vi "UTIL Initialize Median Filter.vi"(8 "Error In":errorcluster, 11 "Window Width":i32=60) -> (0 "Error Out":errorcluster, 3 "Average Queue":refnum<queue>)   [LabVIEW 2010]
doc: "Initialize a Moving Window Average routine by creating a fixed-length, Windows-sized Queue of Dbls, and initializing them to 0.\n\nInput:\n Window Size I32, default 10\n Error In\nOutput:\n Average Queue Fixed-length Queue of Dbl\n Error Out"
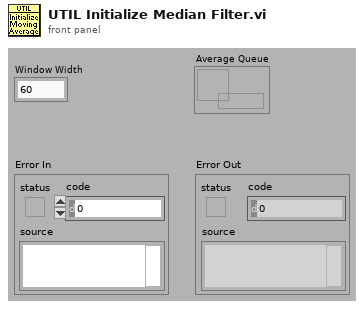
[diagram p1: front panel]
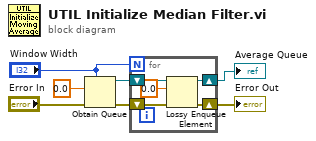
[diagram p0: block diagram]
diagram:
  n1 = Obtain Queue(max queue size (-1, unlimited)="Window Width", element data type=0.0 ("element"), error in (no error)="Error In") -> (queue out=w5:refnum<queue>, error out=w6:errorcluster)  [unwired: 2 in, 1 out]
  n2 = for {
    N: "Window Width" -> [_]
    shift-right: [w11] -> w3
    shift-left: w6 -> [w12]
    shift-right: [w9] -> w1
    shift-left: w5 -> [w10]
    n3 = Lossy Enqueue Element(queue=w10, element=0.0, error in (no error)=w12) -> (queue out=w9:refnum<queue>, error out=w11:errorcluster)  [unwired: 2 out]
  }
  "Error Out" <- w3
  "Average Queue" <- w1
